vi "StateChange.vi"(8 "error in (no error)":errorcluster, 9 "M1M3 Support Events in":refnum<class "M1M3 Support Events.lvclass">, 11 "SAL in":refnum<class "SAL.lvclass">) -> (0 "error out":errorcluster, 3 "SAL out":refnum<class "SAL.lvclass">)   [LabVIEW 2016]
uses:
  SAL.lvclass
  M1M3 Support Events/M1M3 Support Events.lvclass
  M1M3 Support Events/M1M3 Support Events.lvclass/M1M3 Support Events.ctl
  Typedefs/StateTypes.ctl
  Typedefs/M1M3SupportEUI_TypeDefs.lvlib
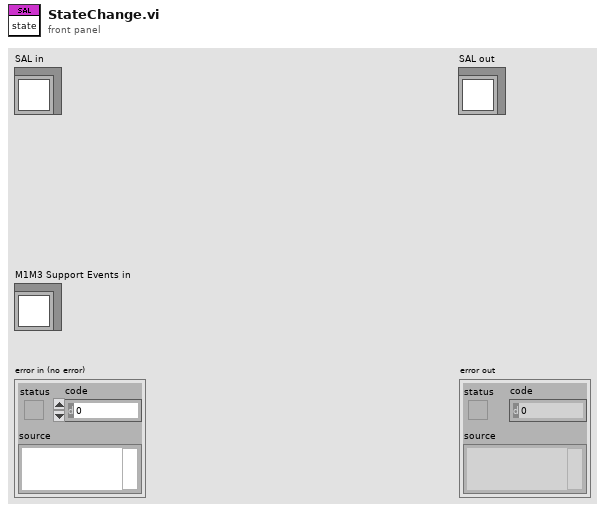
[diagram p1: front panel]
types:
  T1 = typedef "M1M3SupportEUI_TypeDefs.lvlib/M1M3 Support Events.ctl" = cluster{"M1M3 Support State":refnum<user-event>, "Inclinometer  Data":refnum<user-event>, "IMS Data":refnum<user-event>}
  T2 = typedef "M1M3SupportEUI_TypeDefs.lvlib/StateTypes.ctl" = enum16{"Offline State", "Fault State", "Standby State", "Disabled State", "Enabled State", "Wait For User Input State", "Test Actuator State"}
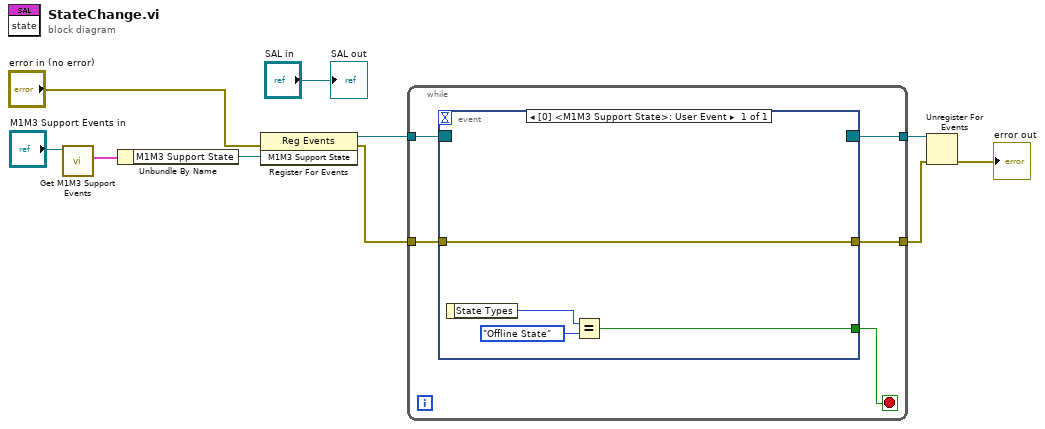
[diagram p0: block diagram]
diagram:
  n1 = call "Get M1M3 Support Events.vi"("M1M3 Support Events in"="M1M3 Support Events in") -> ("M1M3 Support Events"=w8:T1)  [unwired: 9 in, 1 out]
  n2 = Unbundle By Name(w8) -> ("M1M3 Support State"=w7:refnum<user-event>)
  n3 = register-events(error in="error in (no error)", w7) -> (reference out=w6:refnum<event-registration>, error out=w2:errorcluster)  [unwired: 1 in]
  n4 = while {
    tunnel: w6 -> [w15]
    tunnel: [w14] -> w5
    tunnel: w2 -> [w12]
    tunnel: [w11] -> w1
    stop <- w13 stop-if-true
    n5 = event shown="[0] <M1M3 Support State>: User Event" {
      selector: w15 -> [_]
      dyn-events: [_] -> w14
      timeout: _ -> [_]
      tunnel: [w18] -> w13
      tunnel: w12 -> [w16]
      tunnel: [w16] -> w11
      event User Event {
        n6 = event-data() -> ("State Types"=w17:T2)  [unwired: 1 in]
        n7 = Equal?(x=w17, y=StateTypes."Offline State") -> (x = y?=w18:bool)
      }
    }
  }
  n8 = Unregister For Events(event registration refnum=w5, error in=w1) -> (error out=→"error out":errorcluster)
  "SAL out" <- "SAL in"
